vi "Write ForceFollowCycle.vi"(8 "error in (no error)":errorcluster, 10 "ForceFollowCycle":bool, 11 "AI_Snake in":refnum<class "AI_Snake.lvclass">) -> (0 "error out":errorcluster, 3 "AI_Snake out":refnum<class "AI_Snake.lvclass">)   [LabVIEW 2019, in "RT_Game.lvlib" / "AI_Snake.lvclass"]
uses:
  AI_Snake.lvclass
  AI_Snake.lvclass/AI_Snake.ctl
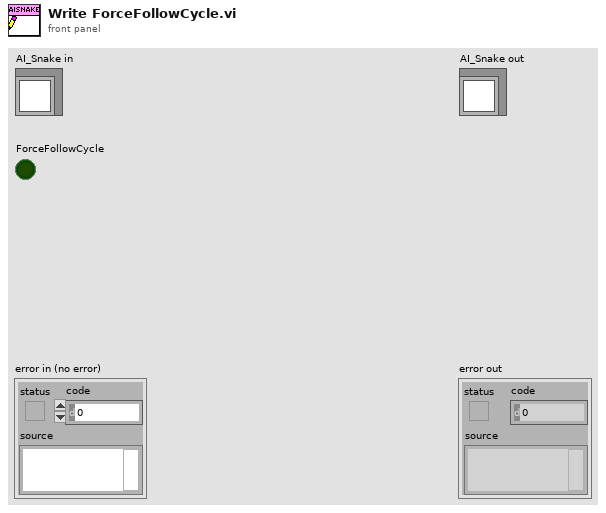
[diagram p1: front panel]
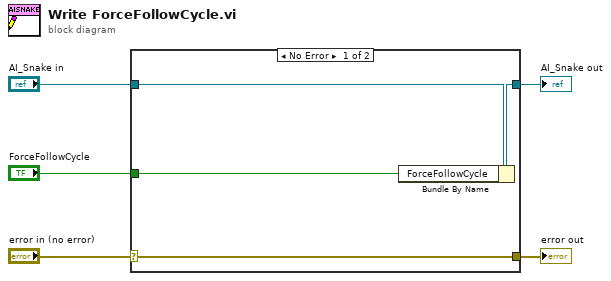
[diagram p0: block diagram]
diagram:
  n1 = case shown="No Error" "error in (no error)" {
    selector: "error in (no error)" -> [w9 w10]
    tunnel: [w9 w10] -> w4
    tunnel: [w7 w11] -> w2
    tunnel: "AI_Snake in" -> [w8 w11]
    tunnel: "ForceFollowCycle" -> [w6 _]
    frame No Error {
      n2 = Bundle By Name(cluster=w8, "ForceFollowCycle"=w6) -> (w7:refnum<class "AI_Snake.lvclass">)
    }
    frame Error {
    }
  }
  "error out" <- w4
  "AI_Snake out" <- w2
